vi "GV1.vi"() -> ()   [LabVIEW 2009]
uses:
  Global 1.vi
panel:
  in  "stop":bool
  in  "data":string
  in  "Expired":bool
  in  "count":dbl
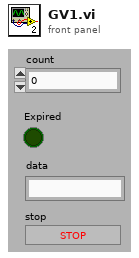
[diagram p1: front panel]
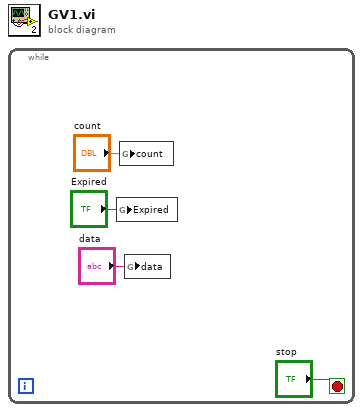
[diagram p0: block diagram]
diagram:
  n1 = while {
    stop <- "stop" stop-if-true
    n2 = global write "Global 1.vi" "Expired"("Expired") -> ()
    n3 = global write "Global 1.vi" "count"("count") -> ()
    n4 = global write "Global 1.vi" "data"("data") -> ()
  }
